vi "SoundMeasure.vi"() -> ()   [LabVIEW 2016]
uses:
  <vilib>/Instr/_visa.llb/VISA Configure Serial Port (Instr).vi
  <vilib>/Utility/config.llb/Read Key (Double).vi
  <vilib>/Utility/file.llb/Write Delimited Spreadsheet (DBL).vi
  <vilib>/Utility/config.llb/NI_LVConfig.lvlib
panel:
  in  "record cycle":u64=7 min=6 step=1
  in  "freq (MHz)":dbl=1.367 min=0.1 max=10.0 step=0.01
  in  "SETVOLT":bool
  out "error out":errorcluster
  in  "cycle":u32=120
  in  "Channel":u16
  in  "KYCT axis in HIFU coordinate":cluster{"X axis":dbl[], "Z axis":dbl[]}={"X axis"=[1.0, 0.0, 0.0], "Z axis"=[0.0, 0.0, 1.0]}
  in  "KYCT coordinate":T1
  in  "Sens (V/MPa)":dbl=0.1
  in  "Port":u32=12321
  in  "HIFU_connect":bool
  in  "HIFU_Telnet":bool
  out "Pressure (MPa)":dbl format="%#_4g"
  in  "pout":bool
  in  "totle chnnum":i16=64
  in  "HIFU IP":string="192.168.1.24"
  in  "SETPHS":bool
  out "XY Graph 2":T2(graph)
  in  "Set global voltage":bool
  in  "Voltage":dbl=4.0 min=0.5 max=20.0 step=1.0
  out "Sonication":bool
  in  "continuousOut":bool
  in  "Scan":bool
  in  "Tab Control":enum32{"1D Scan", "2D Scan", "Monitor"}(tab)
  out "1D plot":cluster{dbl[], dbl[]}(graph)
  out "2D Scan":dbl[][](graph)
  in  "start":bool
  in  "reord":bool
  out "Current":dbl[](graph)
  out "Voltage":dbl[](graph)
  in  "Go":bool
  in  "Speed":dbl=0.5 min=0.2 max=2.5 step=0.1
  in  "Position":dbl[](array[numeric]) format="%#_6f"
  in  "Z+":bool
  in  "Z-":bool
  in  "Y+":bool
  in  "Y-":bool
  in  "X+":bool
  in  "X-":bool
  in  "error in (no error)":errorcluster
  out "HIFU":bool
  out "osc":bool
  out "KYCT":bool
  in  "Exit":bool
  in  "3D motorized stage":refnum<visa-resource-name>
  in  "oscilloscope":refnum<visa-resource-name>
  # "Z"
  # "X"
  # "Y"
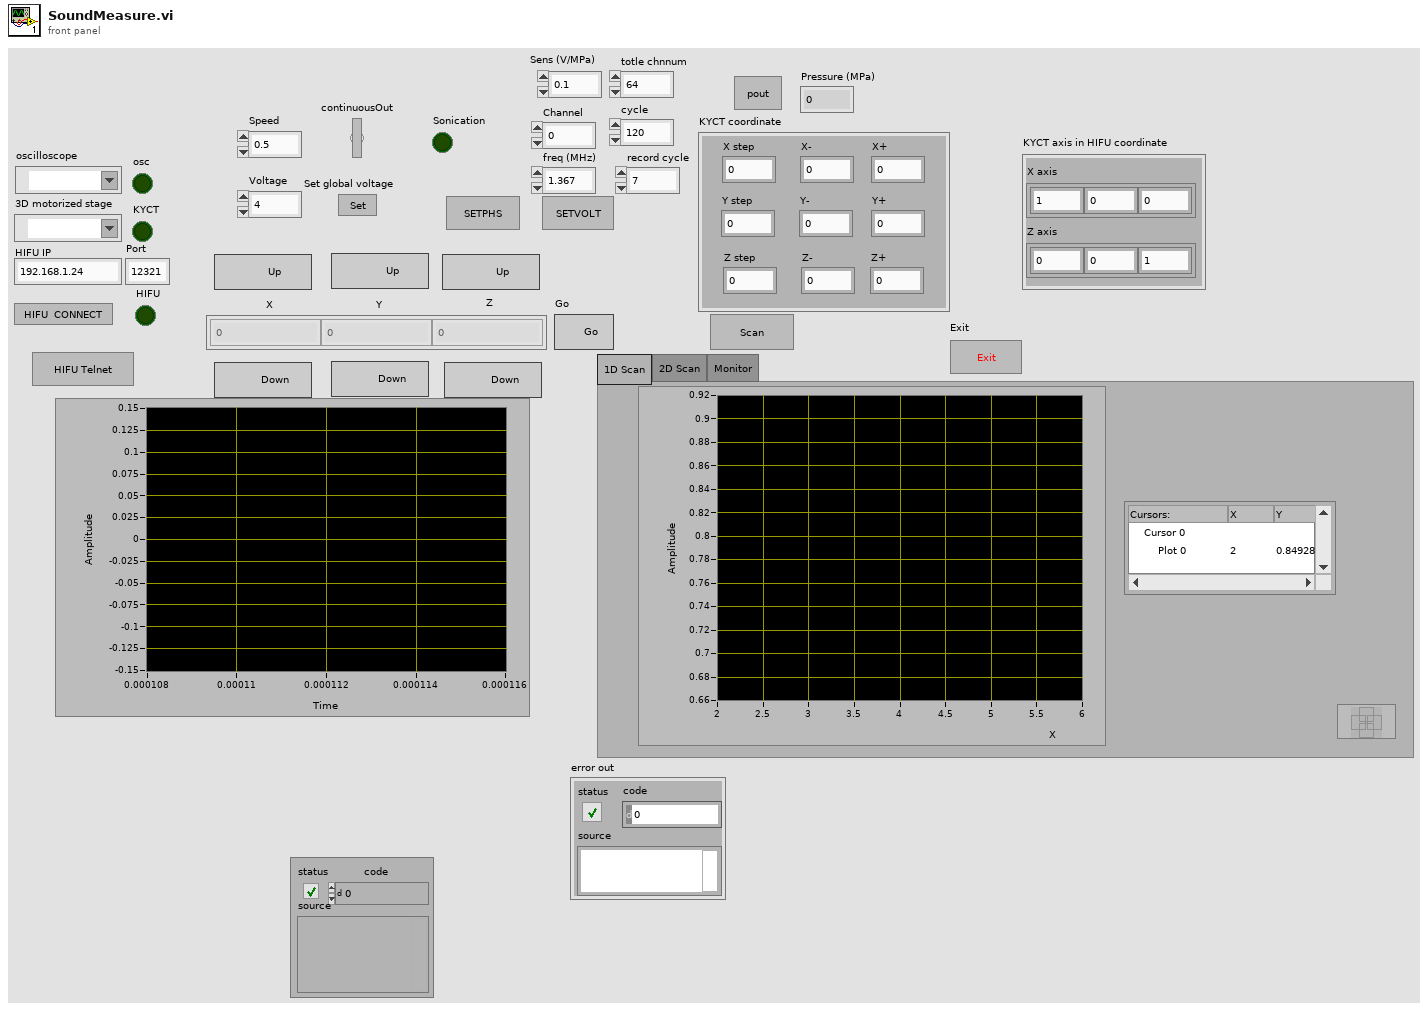
[diagram p1: front panel]
types:
  T1 = cluster{"X-":dbl, "X step":dbl, "Y-":dbl, "Y step":dbl, "Z-":dbl, "Z step":dbl, "Z+":dbl, "X+":dbl, "Y+":dbl}
  T2 = cluster{"time sequence":dbl[], "Voltage sequence":dbl[]}
  T3 = enum8{"Enabled", "Disabled", "Disabled and Grayed Out"}
  T4 = typedef "NI_LVConfig.lvlib/Config Data RefNum.ctl" = refnum<k1>
  T5 = typedef "NI_Matrix.lvlib/RealMatrix.ctl" = dbl[][]
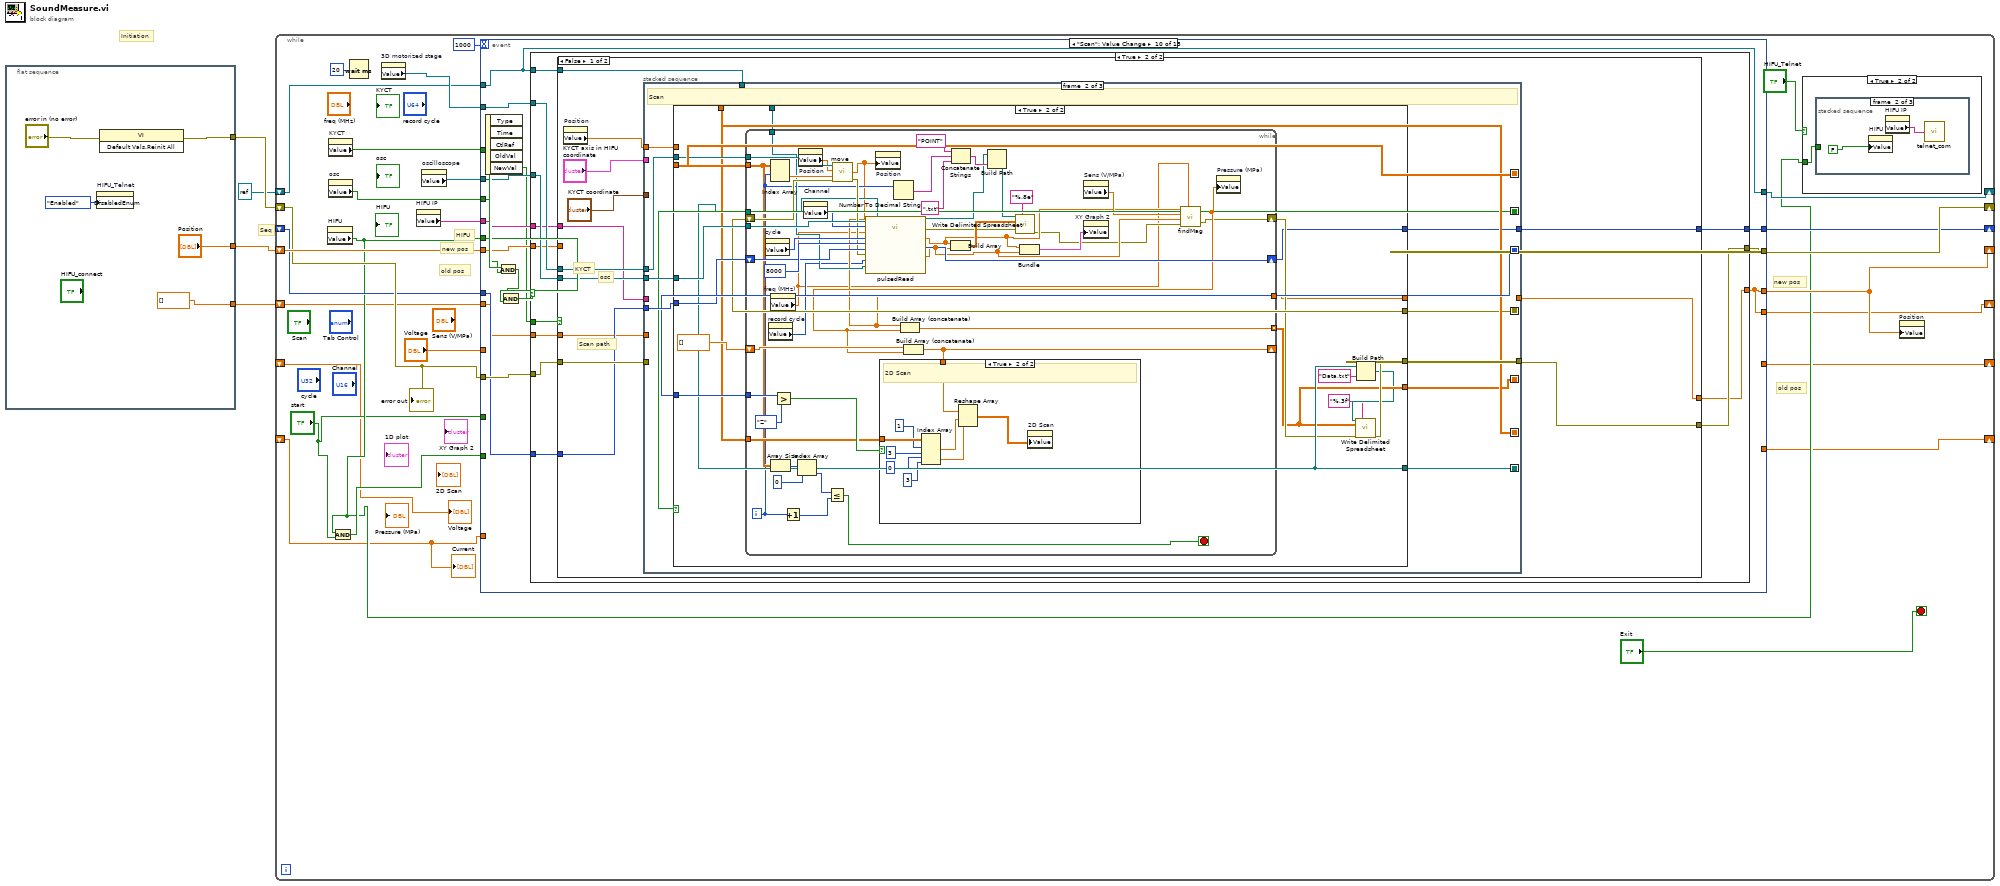
[diagram p0: block diagram]
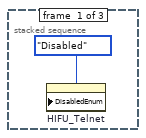
[diagram p3: hidden frame]
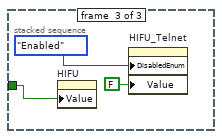
[diagram p4: hidden frame]
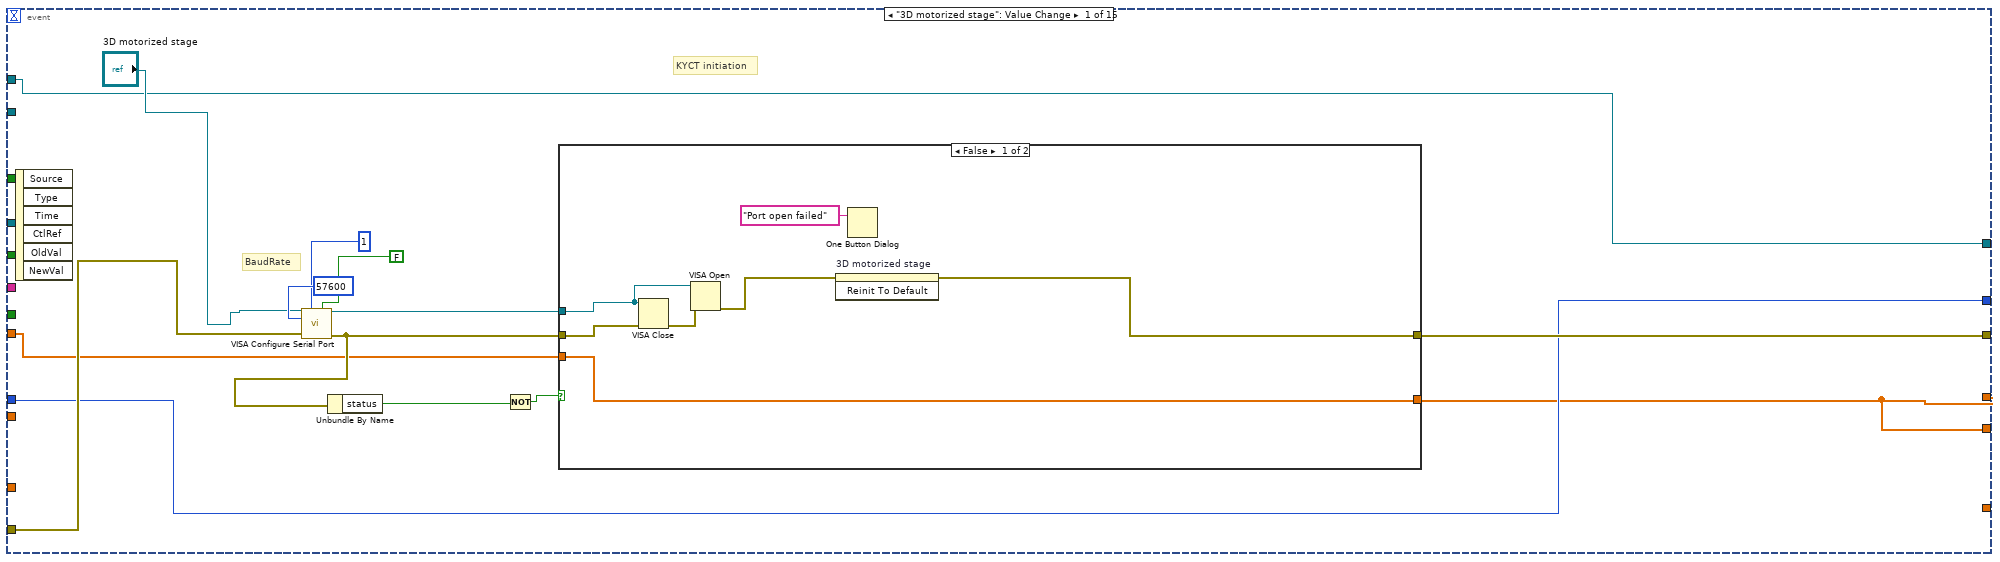
[diagram p5: hidden frame]
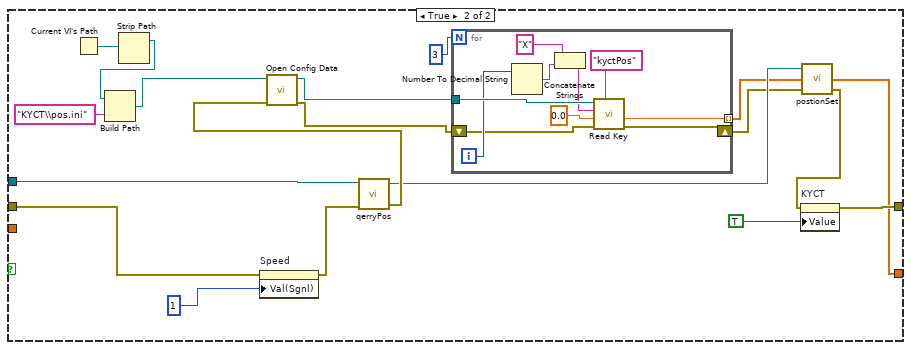
[diagram p6: hidden frame]
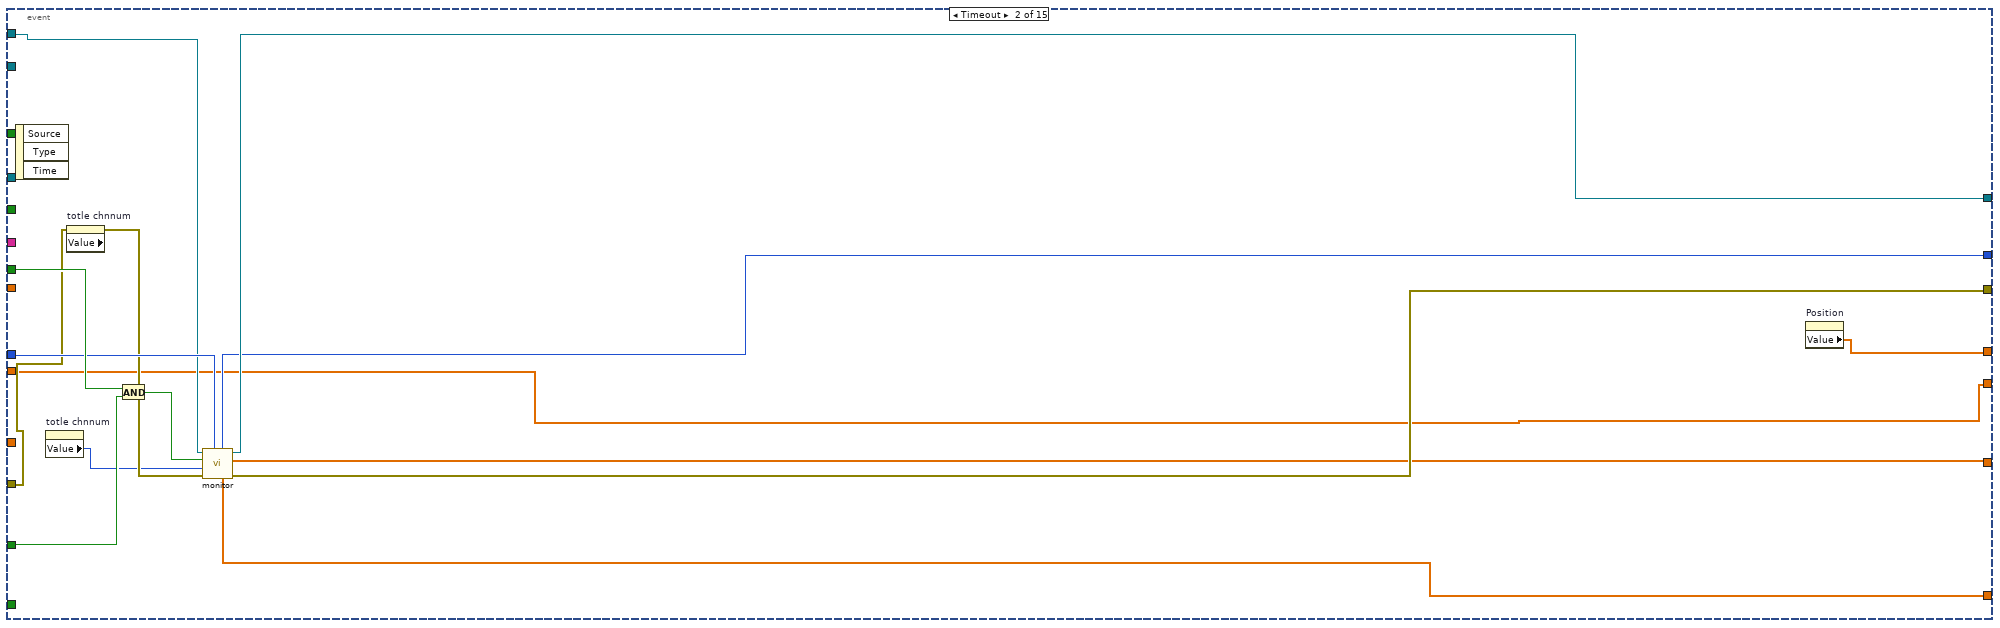
[diagram p7: hidden frame]
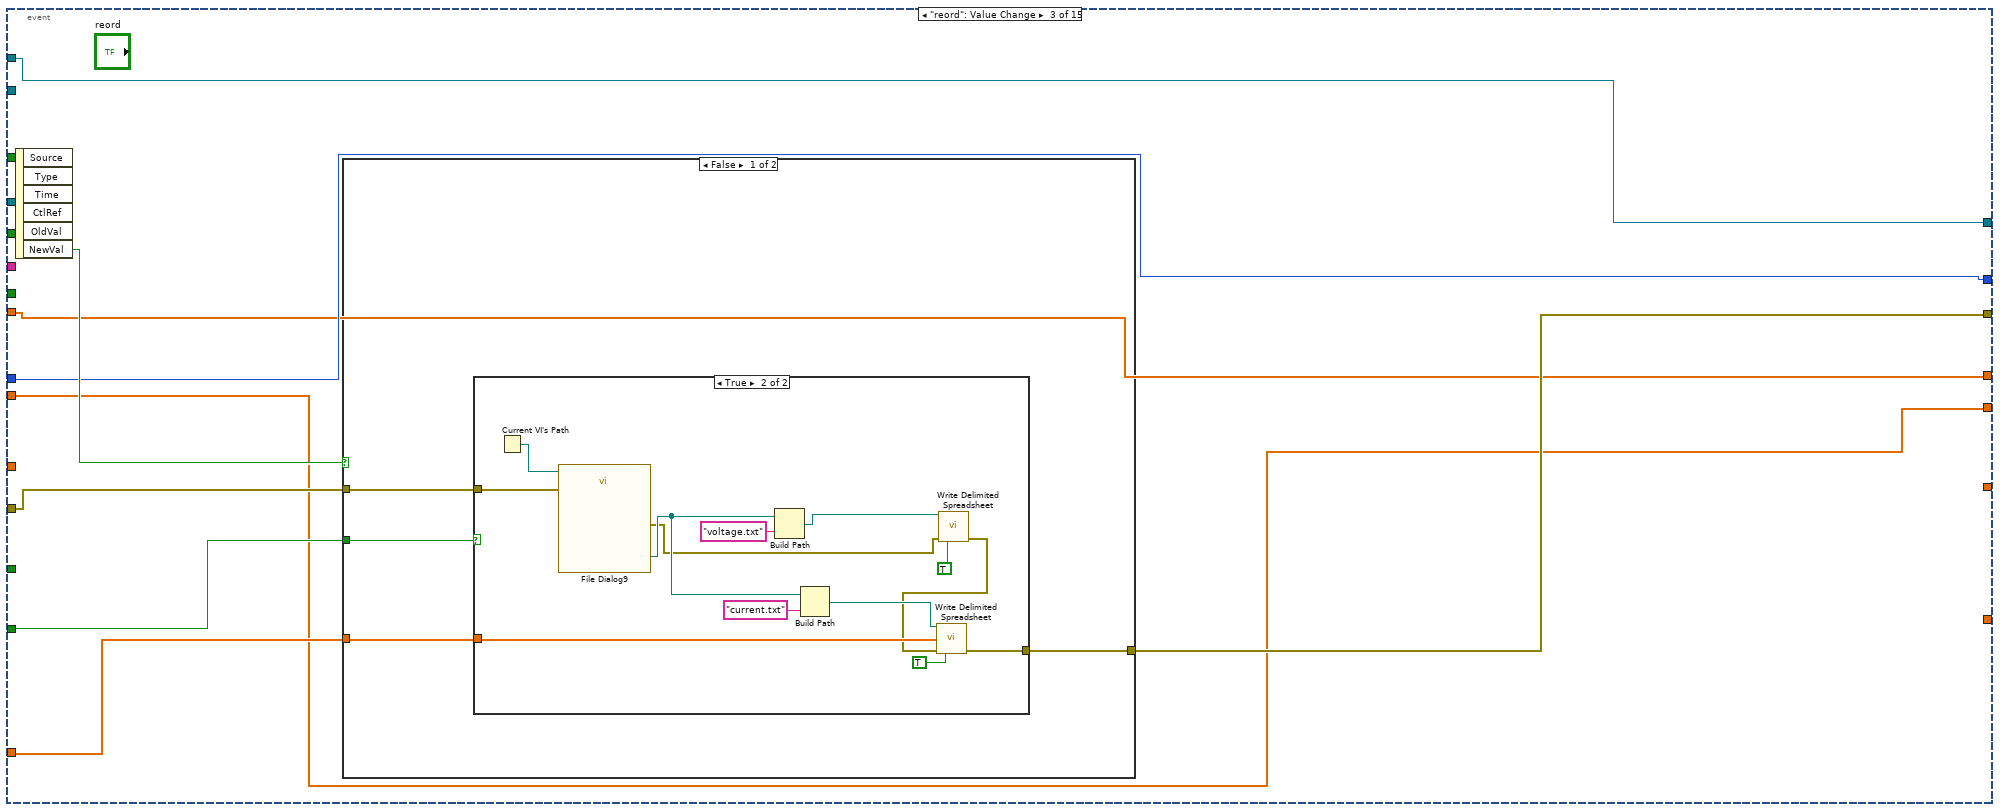
[diagram p8: hidden frame]
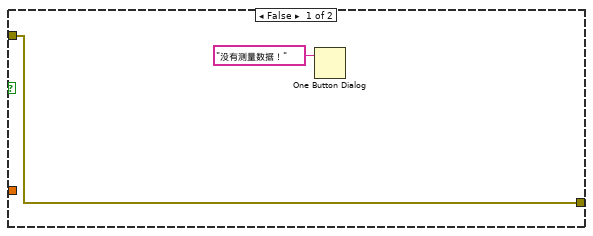
[diagram p9: hidden frame]
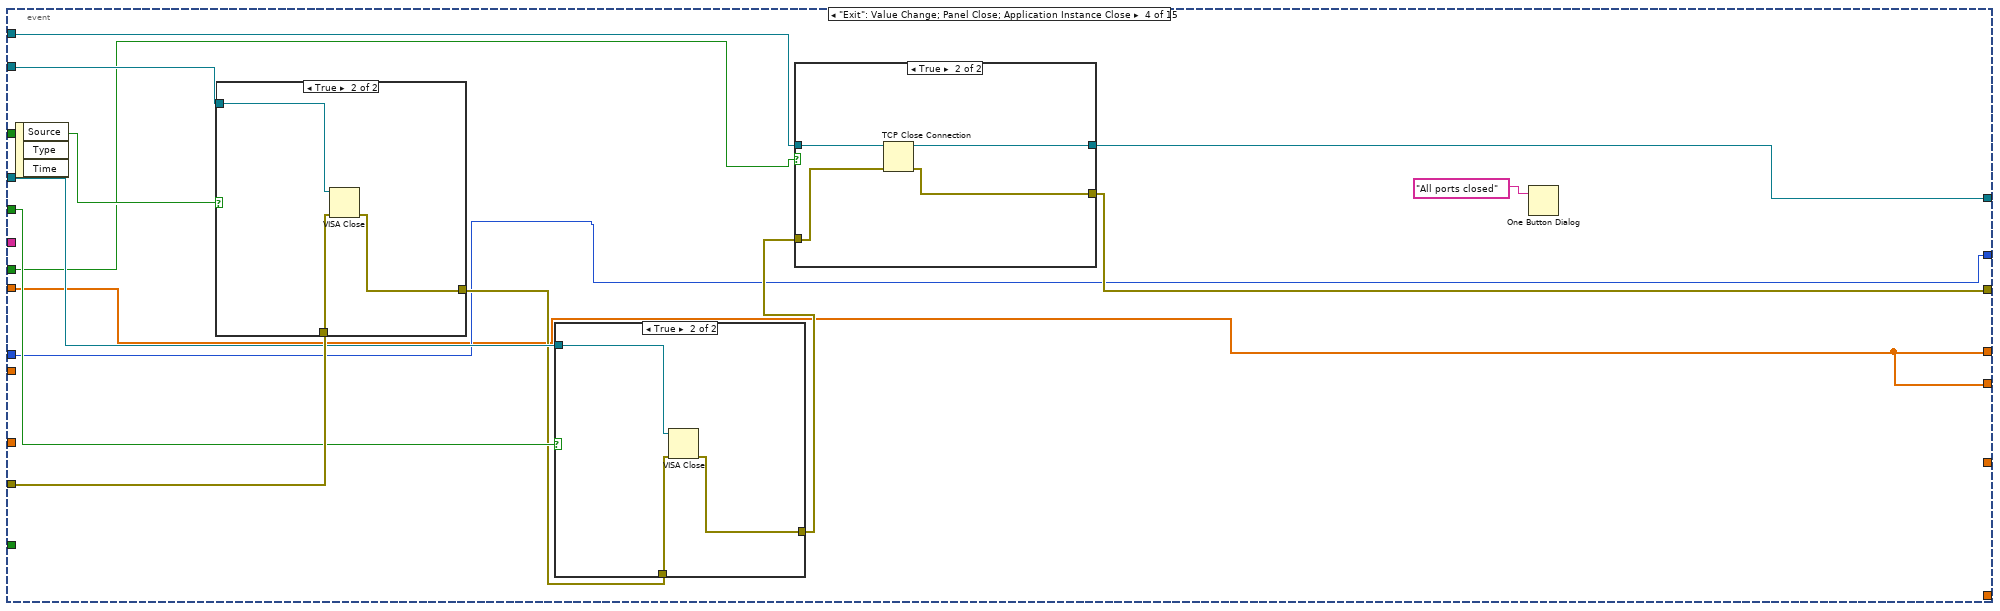
[diagram p11: hidden frame]
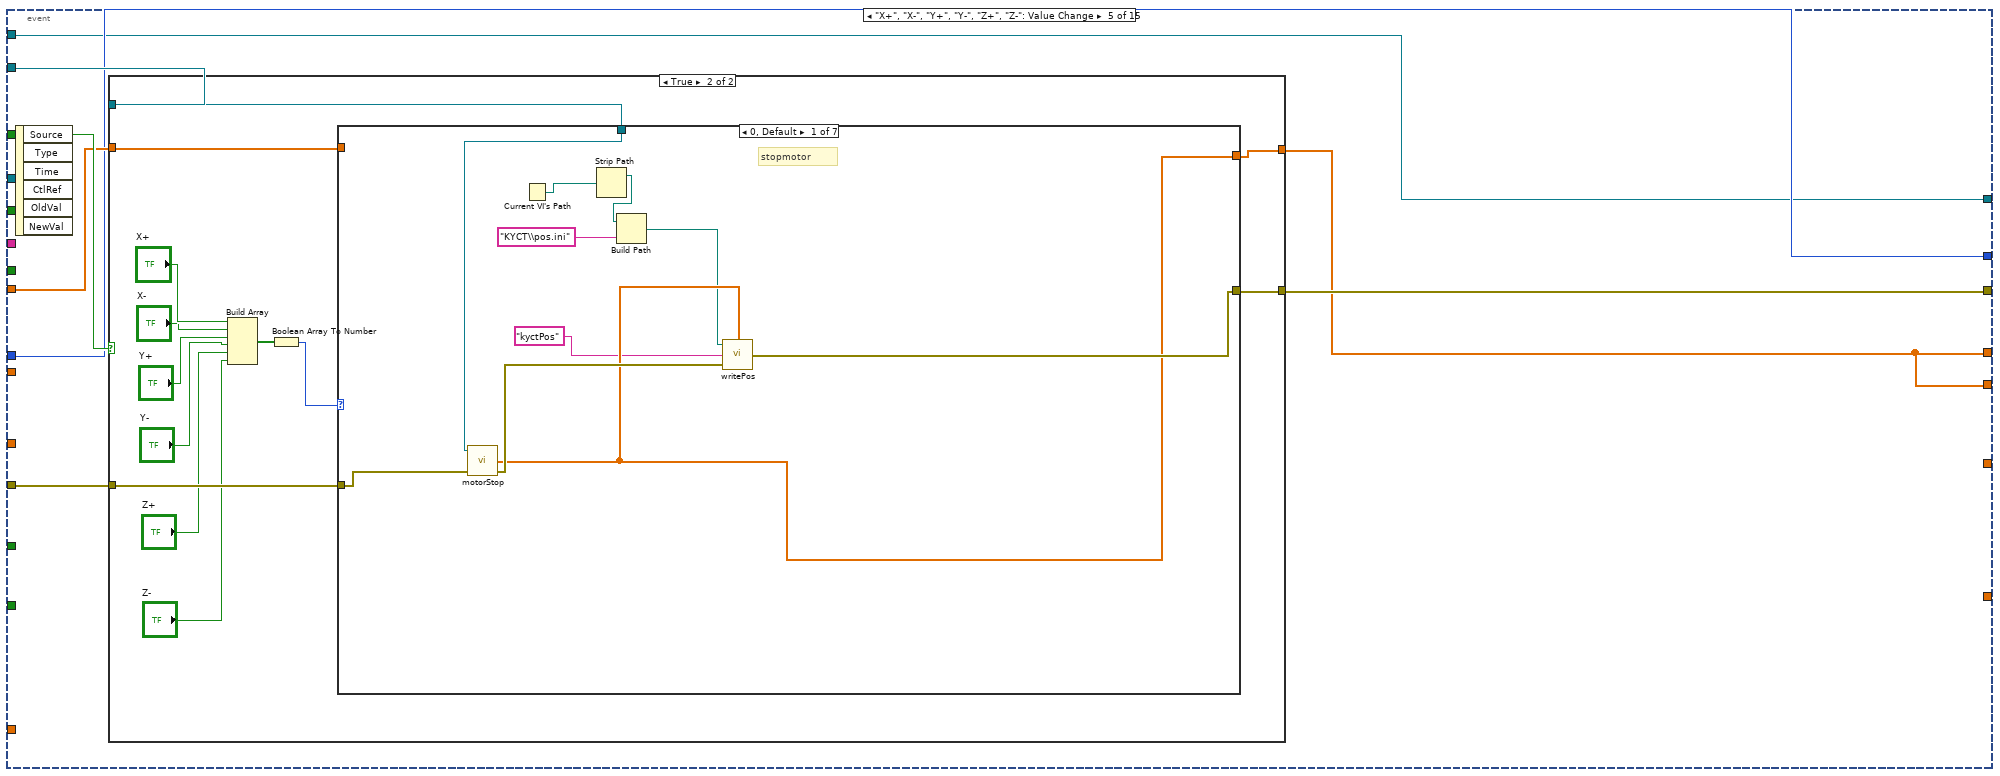
[diagram p15: hidden frame]
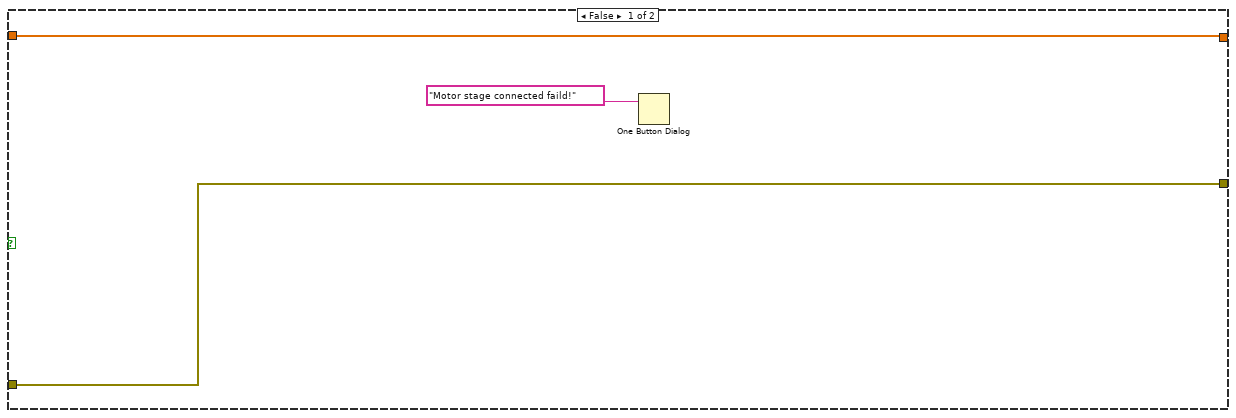
[diagram p16: hidden frame]
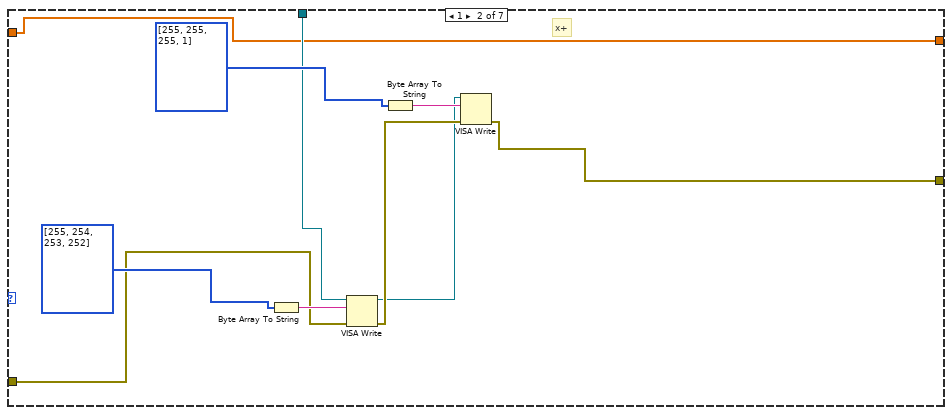
[diagram p17: hidden frame]
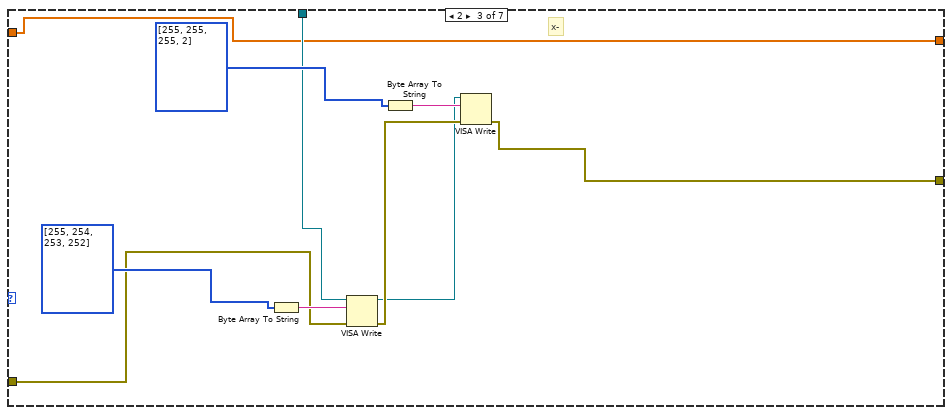
[diagram p18: hidden frame]
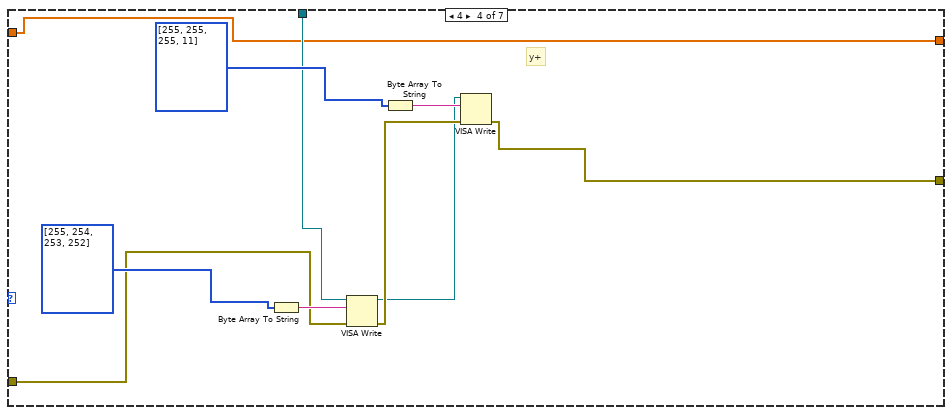
[diagram p19: hidden frame]
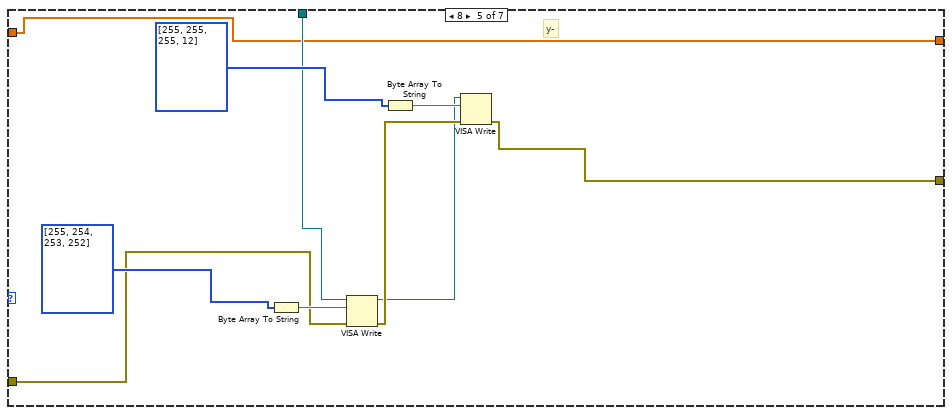
[diagram p20: hidden frame]
diagram:
  # "Seq"
  # "Initiation"
  n1 = flat-sequence {
    tunnel: ["Position"] -> w4
    tunnel: [w8] -> w3
    tunnel: [dbl[] []] -> w1
    frame #0 {
      n2 = property on="HIFU_Telnet" class="Bool (strict)"("DisabledEnum"=T3."Enabled" ("Disabled")) -> ()  [unwired: 2 in, 2 out]
      n3 = invoke class="VI" method="Default Vals.Reinit All"(error in="error in (no error)") -> (error out=w8:errorcluster)  [unwired: 2 in, 2 out]
    }
  }
  n4 = while {
    shift-right: [w34] -> _
    shift-left: w4 -> [w33]
    shift-right: [w32] -> _
    shift-left: w3 -> [w20]
    shift-right: [w23] -> _
    shift-left: refnum<k5> refnum ("connection ID out") -> [w22]
    shift-right: [w21] -> _
    shift-left: _ -> [w19]
    shift-right: [w17] -> _
    shift-left: _ -> [w16]
    shift-right: [w13] -> _
    shift-left: w1 -> [w12]
    shift-right: [w11] -> _
    shift-left: _ -> [w10]
    stop <- "Exit" stop-if-true
    # "HIFU"
    # "old pos"
    # "new pos"
    # "old pos"
    # "new pos"
    n5 = property on="HIFU" class="Bool (strict)"() -> ("Value"=w18:bool)  [unwired: 2 in, 2 out]
    n6 = property on="KYCT" class="Bool (strict)"() -> ("Value"=w36:bool)  [unwired: 2 in, 2 out]
    n7 = property on="osc" class="Bool (strict)"() -> ("Value"=w35:bool)  [unwired: 2 in, 2 out]
    n8 = And(x=w18, y="start") -> (x .and. y?=w25:bool)
    n9 = Wait (ms)(milliseconds to wait=u32 20) -> ()  [unwired: 1 out]
    n10 = property on="3D motorized stage" class="VISAName"() -> ("Value"=w30:refnum<visa-resource-name>)  [unwired: 2 in, 2 out]
    n11 = property on="HIFU IP" class="Str"() -> ("Value"=w26:string)  [unwired: 2 in, 2 out]
    n12 = property on="oscilloscope" class="VISAName"() -> ("Value"=w29:refnum<visa-resource-name>)  [unwired: 2 in, 2 out]
    n13 = event shown="[9] \"Scan\": Value Change" {
      selector: _ -> [_ _ _ _ _ _ _ _ _ _ _ _ _ _ _]
      dyn-events: _ -> [_ _ _ _ _ _ _ _ _ _ _ _ _ _ _]
      timeout: 1000 -> [_ _ _ _ _ _ _ _ _ _ _ _ _ _ _]
      tunnel: w30 -> [_ _ _ w150 w172 w267 w287 _ _ w403 _ _ _ _ _]
      tunnel: w29 -> [_ _ _ w147 _ _ _ _ _ w401 w638 _ _ _ _]
      tunnel: w20 -> [w53 w106 w117 w149 w171 w268 w286 w317 w358 w402 w637 w673 w683 w722 w752]
      tunnel: w36 -> [_ _ _ w151 w173 w266 w288 _ _ w408 _ _ _ _ w756]
      tunnel: [w55 w98 w115 w141 w170 w264 w284 w315 w356 w400 w636 w672 w681 w721 w751] -> w32
      tunnel: w35 -> [_ _ _ w148 _ _ _ _ _ w407 w635 _ _ _ _]
      tunnel: w33 -> [w48 _ w110 w138 w169 w261 _ w318 w359 w399 w639 w674 w684 w719 w755]
      tunnel: [w44 w96 w110 w138 w166 w261 w279 w318 w359 w393 w639 w674 w684 w719 w754] -> w34
      tunnel: w18 -> [_ w108 _ w144 _ _ _ w316 w357 w406 w634 _ _ w718 w749]
      tunnel: "Voltage" -> [_ _ _ _ _ _ _ _ _ _ _ _ _ w720 _]
      tunnel: w16 -> [_ _ w116 _ _ _ _ _ _ _ _ _ _ _ _]
      tunnel: w26 -> [_ _ _ _ _ _ _ _ _ w398 _ _ _ _ w748]
      tunnel: w25 -> [_ _ w114 _ _ _ _ _ _ _ _ _ _ _ _]
      tunnel: [w46 w102 w112 w139 w167 w262 w281 w313 w354 w394 w629 w669 w679 w714 w744] -> w23
      tunnel: w22 -> [w46 w103 w112 w142 w167 w262 w281 w313 w354 w394 w629 w669 _ w714 w747]
      tunnel: [w45 w100 w111 w140 w168 w263 w282 w311 w352 w395 w630 w670 w678 w715 w745] -> w21
      tunnel: w19 -> [w45 w107 w111 w140 w168 w263 w282 w312 w353 w396 w631 w670 _ w716 w746]
      tunnel: [_ w101 _ _ _ _ _ _ _ _ _ _ _ _ _] -> w17
      tunnel: "start" -> [_ w99 _ _ _ _ _ _ _ _ _ _ _ _ _]
      tunnel: [w44 w95 w109 w138 w166 w260 w278 w310 w351 w393 w628 w668 w677 w713 w743] -> w13
      tunnel: w12 -> [_ w95 w109 _ _ w260 w280 w310 w351 w392 w628 w668 w677 w713 w743]
      tunnel: [_ w94 _ _ _ _ _ _ _ _ _ _ _ _ _] -> w11
      event "3D motorized stage": Value Change {
        # "KYCT initiation"
        # "BaudRate"
        n14 = event-data() -> ()  [unwired: 1 in, 6 out]
        n15 = call-poly "VISA Configure Serial Port"("VISA resource name"="3D motorized stage", "timeout (10sec)"=u32 1, "Enable Termination\nChar (T)"=FALSE, "baud rate (9600)"=u32 57600, "error in (no error)"=w53) -> ("VISA resource name out"=w56:refnum<visa-resource-name>, "error out"=w51:errorcluster)  [unwired: 9 in]
        n16 = Unbundle By Name(w51) -> ("status"=w50:bool)
        n17 = Not(x=w50) -> (.not. x?=w49:bool)
        n18 = case shown="False" w49 {
          tunnel: w56 -> [w58 w81]
          tunnel: [w64 w66] -> w44
          tunnel: [w63 w80] -> w55
          tunnel: w51 -> [w61 w78]
          tunnel: w48 -> [w64 _]
          frame False {
            n19 = VISA Close(VISA resource name=w58, error in (no error)=w61) -> (error out=w60:errorcluster)
            n20 = VISA Open(error in (no error)=w60, VISA resource name=w58) -> (error out=w59:errorcluster)  [unwired: 3 in, 1 out]
            n21 = invoke on="3D motorized stage" class="VISAName" method="Reinit To Default"(error in=w59) -> (error out=w63:errorcluster)  [unwired: 2 in, 2 out]
            n22 = One Button Dialog(message="Port open failed") -> ()  [unwired: 1 in, 1 out]
          }
          frame True {
            n23 = Current VI's Path() -> (path=w77:path)
            n24 = Strip Path(path=w77) -> (stripped path=w76:path)  [unwired: 1 out]
            n25 = Build Path(base path=w76, name or relative path="KYCT\\pos.ini") -> (appended path=w74:path)
            n26 = property on="Speed" class="DigNum (strict)"(error in=w78, "Val(Sgnl)"=1) -> (error out=w79:errorcluster)  [unwired: 1 in, 1 out]
            n27 = call "qerryPos.vi"("error in (no error)"=w79, "UART in"=w81) -> ("error out"=w73:errorcluster, "UART out"=w69:refnum<visa-resource-name>)  [unwired: 2 in, 1 out]
            n28 = call <vilib>:"Open Config Data.vi"("error in (no error)"=w73, "configuration file path"=w74) -> ("error out"=w71:errorcluster, "refnum"=w70:T4)  [unwired: 7 in, 1 out]
            n29 = for {
              N: 3 -> [_]
              tunnel: w70 -> [w93]
              shift-right: [w86] -> w68
              shift-left: w71 -> [w87]
              tunnel: [w85] -> w67 mode=indexing
              i -> [w89]
              n30 = Number To Decimal String(number=w89) -> (decimal integer string=w91:string)  [unwired: 1 in]
              n31 = Concatenate Strings("X" ("string"), w91) -> (w90:string)
              n32 = call-poly <vilib>:"Read Key.vi"("section"="kyctPos", "error in (no error)"=w87, "default value"=0.0, "key"=w90, "refnum"=w93) -> ("error out"=w86:errorcluster, "value"=w85:dbl)  [unwired: 3 in, 2 out]
            }
            n33 = call "postionSet.vi"("error in (no error)"=w68, "Pos in"=w67, "UART PORT in"=w69) -> ("error out"=w65:errorcluster, "Pos out"=w66:dbl[])  [unwired: 1 out]
            n34 = property on="KYCT" class="Bool (strict)"(error in=w65, "Value"=TRUE) -> (error out=w80:errorcluster)  [unwired: 1 in, 1 out]
          }
        }
      }
      event Timeout {
        n35 = event-data() -> ()  [unwired: 1 in, 3 out]
        n36 = property on="totle chnnum" class="DigNum (strict)"() -> ("Value"=w97:i16)  [unwired: 2 in, 2 out]
        n37 = property on="totle chnnum" class="DigNum (strict)" props=["Value"](error in=w106) -> (error out=w105:errorcluster)  [unwired: 1 in, 2 out]
        n38 = And(x=w108, y=w99) -> (x .and. y?=w104:bool)
        n39 = call "monitor.vi"("HIFU_TCP in"=w103, "HIFU"=w104, "chn num"=w97, "error in (no error)"=w105, "sequence"=w107) -> ("SEQ out"=w100:u32, "current"=w101:dbl[], "HIFU_TCP out"=w102:refnum<k5>, "voltage"=w94:dbl[], "error out"=w98:errorcluster)  [unwired: 1 out]
        n40 = property on="Position" class="Arr (strict)"() -> ("Value"=w96:dbl[])  [unwired: 2 in, 2 out]
      }
      event "reord": Value Change {
        n41 = event-data() -> ("NewVal"=w113:bool)  [unwired: 1 in, 5 out]
        n42 = case shown="False" w113 {
          tunnel: w117 -> [w121 w137]
          tunnel: w116 -> [w120 _]
          tunnel: [w119 w137] -> w115
          tunnel: w114 -> [w118 _]
          frame False {
            n43 = case shown="True" w118 {
              tunnel: w121 -> [w123 w131]
              tunnel: w120 -> [_ w128]
              tunnel: [w123 w126] -> w119
              frame False {
                n44 = One Button Dialog(message="没有测量数据！") -> ()  [unwired: 1 in, 1 out]
              }
              frame True {
                n45 = Current VI's Path() -> (path=w136:path)
                n46 = call "File Dialog9"("start path"=w136, "error in"=w131) -> ("selected path"=w133:path, "error out"=w130:errorcluster)  [unwired: 10 in, 2 out]
                n47 = Build Path(base path=w133, name or relative path="voltage.txt") -> (appended path=w132:path)
                n48 = Build Path(base path=w133, name or relative path="current.txt") -> (appended path=w129:path)
                n49 = call-poly <vilib>:"Write Delimited Spreadsheet.vi"("file path (dialog if empty)"=w132, "error in (no error)"=w130, "transpose? (no:F)"=TRUE) -> ("error out"=w127:errorcluster)  [unwired: 11 in, 1 out]
                n50 = call-poly <vilib>:"Write Delimited Spreadsheet.vi"("file path (dialog if empty)"=w129, "1D data"=w128, "error in (no error)"=w127, "transpose? (no:F)"=TRUE) -> ("error out"=w126:errorcluster)  [unwired: 10 in, 1 out]
              }
            }
          }
          frame True {
          }
        }
      }
      event "Exit": Value Change; Panel Close; Application Instance Close {
        n51 = event-data() -> ()  [unwired: 1 in, 3 out]
        n52 = case shown="True" w151 {
          tunnel: w150 -> [_ w165]
          tunnel: w149 -> [w162 w164]
          tunnel: [w162 w163] -> w146
          frame False {
          }
          frame True {
            n53 = VISA Close(VISA resource name=w165, error in (no error)=w164) -> (error out=w163:errorcluster)
          }
        }
        n54 = case shown="True" w148 {
          tunnel: w147 -> [_ w161]
          tunnel: w146 -> [w158 w160]
          tunnel: [w158 w159] -> w143
          frame False {
          }
          frame True {
            n55 = VISA Close(VISA resource name=w161, error in (no error)=w160) -> (error out=w159:errorcluster)
          }
        }
        n56 = case shown="True" w144 {
          tunnel: w143 -> [w153 w156]
          tunnel: w142 -> [w152 w157]
          tunnel: [w153 w155] -> w141
          tunnel: [w152 w154] -> w139
          frame False {
          }
          frame True {
            n57 = TCP Close Connection(connection ID=w157, error in (no error)=w156) -> (connection ID out=w154:refnum<k5>, error out=w155:errorcluster)  [unwired: 1 in]
          }
        }
        n58 = One Button Dialog(message="All ports closed") -> ()  [unwired: 1 in, 1 out]
      }
      event "X+", "X-", "Y+", "Y-", "Z+", "Z-": Value Change {
        n59 = event-data() -> ()  [unwired: 1 in, 6 out]
        n60 = case shown="True" w173 {
          tunnel: w172 -> [_ w188]
          tunnel: w171 -> [w175 w189]
          tunnel: [w175 w187] -> w170
          tunnel: [w174 w185] -> w166
          tunnel: w169 -> [w174 w186]
          frame False {
            n61 = One Button Dialog(message="Motor stage connected faild!") -> ()  [unwired: 1 in, 1 out]
          }
          frame True {
            n62 = Build Array("X+", "X-", "Y+", "Y-", "Z+", "Z-") -> (w178:bool[])
            n63 = Boolean Array To Number(Boolean array=w178) -> (number=w177:u32)
            n64 = case shown="0, Default" w177 {
              tunnel: w189 -> [w199 w205 w215 w225 w235 w245 w255]
              tunnel: w188 -> [w198 w204 w214 w224 w234 w244 w254]
              tunnel: [w196 w201 w211 w221 w231 w241 w251] -> w187
              tunnel: w186 -> [_ w200 w210 w220 w230 w240 w250]
              tunnel: [w195 w200 w210 w220 w230 w240 w250] -> w185
              frame 0, Default {
                # "stopmotor"
                n65 = call "motorStop.vi"("error in (no error)"=w199, "UART PORT in"=w198) -> ("error out"=w197:errorcluster, "P1"=w195:dbl[])  [unwired: 1 in, 1 out]
                n66 = Current VI's Path() -> (path=w193:path)
                n67 = Strip Path(path=w193) -> (stripped path=w192:path)  [unwired: 1 out]
                n68 = Build Path(base path=w192, name or relative path="KYCT\\pos.ini") -> (appended path=w191:path)
                n69 = call "writePos.vi"("Pos"=w195, "error in (no error)"=w197, "name"="kyctPos", "ini Path in"=w191) -> ("error out"=w196:errorcluster)
              }
              frame 1 {
                # "x+"
                n70 = Byte Array To String(unsigned byte array=i32[] [255, 254, 253, 252]) -> (string=w207:string)
                n71 = VISA Write(VISA resource name=w204, write buffer=w207, error in (no error)=w205) -> (VISA resource name out=w202:refnum<visa-resource-name>, error out=w203:errorcluster)  [unwired: 1 out]
                n72 = Byte Array To String(unsigned byte array=i32[] [255, 255, 255, 1]) -> (string=w209:string)
                n73 = VISA Write(VISA resource name=w202, write buffer=w209, error in (no error)=w203) -> (error out=w201:errorcluster)  [unwired: 2 out]
              }
              frame 2 {
                # "x-"
                n74 = Byte Array To String(unsigned byte array=i32[] [255, 254, 253, 252]) -> (string=w217:string)
                n75 = VISA Write(VISA resource name=w214, write buffer=w217, error in (no error)=w215) -> (VISA resource name out=w212:refnum<visa-resource-name>, error out=w213:errorcluster)  [unwired: 1 out]
                n76 = Byte Array To String(unsigned byte array=i32[] [255, 255, 255, 2]) -> (string=w219:string)
                n77 = VISA Write(VISA resource name=w212, write buffer=w219, error in (no error)=w213) -> (error out=w211:errorcluster)  [unwired: 2 out]
              }
              frame 4 {
                # "y+"
                n78 = Byte Array To String(unsigned byte array=i32[] [255, 254, 253, 252]) -> (string=w227:string)
                n79 = VISA Write(VISA resource name=w224, write buffer=w227, error in (no error)=w225) -> (VISA resource name out=w222:refnum<visa-resource-name>, error out=w223:errorcluster)  [unwired: 1 out]
                n80 = Byte Array To String(unsigned byte array=i32[] [255, 255, 255, 11]) -> (string=w229:string)
                n81 = VISA Write(VISA resource name=w222, write buffer=w229, error in (no error)=w223) -> (error out=w221:errorcluster)  [unwired: 2 out]
              }
              frame 8 {
                # "y-"
                n82 = Byte Array To String(unsigned byte array=i32[] [255, 254, 253, 252]) -> (string=w237:string)
                n83 = VISA Write(VISA resource name=w234, write buffer=w237, error in (no error)=w235) -> (VISA resource name out=w232:refnum<visa-resource-name>, error out=w233:errorcluster)  [unwired: 1 out]
                n84 = Byte Array To String(unsigned byte array=i32[] [255, 255, 255, 12]) -> (string=w239:string)
                n85 = VISA Write(VISA resource name=w232, write buffer=w239, error in (no error)=w233) -> (error out=w231:errorcluster)  [unwired: 2 out]
              }
              frame 16 {
                # "z+"
                n86 = Byte Array To String(unsigned byte array=i32[] [255, 254, 253, 252]) -> (string=w247:string)
                n87 = VISA Write(VISA resource name=w244, write buffer=w247, error in (no error)=w245) -> (VISA resource name out=w242:refnum<visa-resource-name>, error out=w243:errorcluster)  [unwired: 1 out]
                n88 = Byte Array To String(unsigned byte array=i32[] [255, 255, 255, 21]) -> (string=w249:string)
                n89 = VISA Write(VISA resource name=w242, write buffer=w249, error in (no error)=w243) -> (error out=w241:errorcluster)  [unwired: 2 out]
              }
              frame 32 {
                # "z-"
                n90 = Byte Array To String(unsigned byte array=i32[] [255, 254, 253, 252]) -> (string=w257:string)
                n91 = VISA Write(VISA resource name=w254, write buffer=w257, error in (no error)=w255) -> (VISA resource name out=w252:refnum<visa-resource-name>, error out=w253:errorcluster)  [unwired: 1 out]
                n92 = Byte Array To String(unsigned byte array=i32[] [255, 255, 255, 22]) -> (string=w259:string)
                n93 = VISA Write(VISA resource name=w252, write buffer=w259, error in (no error)=w253) -> (error out=w251:errorcluster)  [unwired: 2 out]
              }
            }
          }
        }
      }
      event "Speed": Value Change {
        n94 = event-data() -> ()  [unwired: 1 in, 6 out]
        n95 = case shown="False" w266 {
          tunnel: "Speed" -> [_ w276]
          tunnel: w268 -> [w270 w275]
          tunnel: w267 -> [_ w274]
          tunnel: [w270 w271] -> w264
          frame False {
            n96 = One Button Dialog(message="Motor stage connected faild!") -> ()  [unwired: 1 in, 1 out]
          }
          frame True {
            n97 = call "setVel.vi"("error in (no error)"=w275, "speed"=w276, "UART in"=w274) -> ("error out"=w273:errorcluster, "UART out"=w272:refnum<visa-resource-name>)
            n98 = property on="3D motorized stage" class="VISAName"(error in=w273, "Value"=w272) -> (error out=w271:errorcluster)  [unwired: 1 in, 1 out]
          }
        }
      }
      event "Go": Value Change {
        n99 = event-data() -> ("NewVal"=w283:bool)  [unwired: 1 in, 5 out]
        n100 = property on="Position" class="Arr (strict)"() -> ("Value"=w277:dbl[])  [unwired: 2 in, 2 out]
        n101 = case shown="True" w288 {
          tunnel: w287 -> [_ w300]
          tunnel: w286 -> [w291 w299]
          tunnel: [w290 w295] -> w279
          tunnel: [w291 w298] -> w285
          tunnel: w277 -> [w290 w296]
          tunnel: w283 -> [_ w297]
          tunnel: w280 -> [w289 w294]
          tunnel: [w289 w293] -> w278
          frame False {
            n102 = One Button Dialog(message="Motor stage connected faild!") -> ()  [unwired: 1 in, 1 out]
          }
          frame True {
            n103 = case shown="False" w297 {
              tunnel: w300 -> [w306 _]
              tunnel: w299 -> [w305 w309]
              tunnel: [w304 w309] -> w298
              tunnel: [w301 w308] -> w295
              tunnel: w296 -> [w303 w308]
              tunnel: w294 -> [w302 w307]
              tunnel: [w301 w307] -> w293
              frame False {
                n104 = call "move.vi"("error in (no error)"=w305, "P01"=w303, "P0"=w302, "UART PORT in"=w306) -> ("error out"=w304:errorcluster, "P1"=w301:dbl[])  [unwired: 1 out]
              }
              frame True {
              }
            }
          }
        }
        n105 = invoke on="Go" class="Bool" method="Reinit To Default"(error in=w285) -> (error out=w284:errorcluster)  [unwired: 2 in, 2 out]
      }
      event "SETPHS": Value Change {
        n106 = event-data() -> ("NewVal"=w314:bool)  [unwired: 1 in, 5 out]
        n107 = case shown="True" w316 {
          tunnel: w317 -> [w321 w326]
          tunnel: [w321 w327] -> w315
          tunnel: w314 -> [_ w325]
          tunnel: w313 -> [_ w324]
          tunnel: w312 -> [w319 w323]
          tunnel: [w319 w322] -> w311
          frame False {
            n108 = One Button Dialog(message="i2c connected failed") -> ()  [unwired: 1 in, 1 out]
          }
          frame True {
            n109 = case shown="False" w325 {
              tunnel: [w335 w350] -> w327
              tunnel: w326 -> [w334 w350]
              tunnel: w324 -> [w331 _]
              tunnel: w323 -> [w329 w349]
              tunnel: [w328 w349] -> w322
              frame False {
                n110 = call "File Dialog8"("error in"=w334) -> ("selected path"=w338:path, "error out"=w333:errorcluster)  [unwired: 11 in, 2 out]
                n111 = case shown="No Error" w333 {
                  selector: w333 -> [w339 w345]
                  tunnel: w338 -> [w342 _]
                  tunnel: [w341 w346] -> w337
                  tunnel: [w340 w344] -> w336
                  frame No Error {
                    n112 = call "readPHS.vi"("error in (no error)"=w339, "Path"=w342) -> ("error out"=w340:errorcluster, "Array"=w341:u8[])
                  }
                  frame Error {
                    n113 = call <vilib>:"Clear Errors.vi"("error in (no error)"=w345, "specific error code to clear (0: all)"=43) -> ("error out"=w344:errorcluster)  [unwired: 4 in, 1 out]
                    n114 = for {
                      N: 64 -> [_]
                      tunnel: [0] -> w346 mode=indexing
                    }
                  }
                }
                n115 = call "PhaseSet.vi"("相位输入"=w337, "HIFU"=TRUE, "error in (no error)"=w336, "chn num"="totle chnnum", "SeqNum"=w329, "connection ID in"=w331) -> ("error out"=w335:errorcluster, "SeqOUT"=w328:u32)  [unwired: 2 out]
              }
              frame True {
              }
            }
          }
        }
      }
      event "SETVOLT": Value Change {
        n116 = event-data() -> ("NewVal"=w355:bool)  [unwired: 1 in, 5 out]
        n117 = case shown="True" w357 {
          tunnel: w358 -> [w362 w367]
          tunnel: [w362 w368] -> w356
          tunnel: w355 -> [_ w366]
          tunnel: w354 -> [_ w365]
          tunnel: w353 -> [w360 w364]
          tunnel: [w360 w363] -> w352
          frame False {
            n118 = One Button Dialog(message="i2c connected failed") -> ()  [unwired: 1 in, 1 out]
          }
          frame True {
            n119 = case shown="False" w366 {
              tunnel: [w376 w391] -> w368
              tunnel: w367 -> [w375 w391]
              tunnel: w365 -> [w373 _]
              tunnel: w364 -> [w371 w390]
              tunnel: [w370 w390] -> w363
              frame False {
                n120 = call "File Dialog2"("error in"=w375) -> ("selected path"=w379:path, "error out"=w374:errorcluster)  [unwired: 11 in, 2 out]
                n121 = case shown="No Error" w374 {
                  selector: w374 -> [w380 w386]
                  tunnel: w379 -> [w383 _]
                  tunnel: [w382 w387] -> w378
                  tunnel: [w381 w385] -> w377
                  frame No Error {
                    n122 = call "readVoltFile.vi"("error in (no error)"=w380, "Path"=w383) -> ("error out"=w381:errorcluster, "Array"=w382:sgl[])
                  }
                  frame Error {
                    n123 = call <vilib>:"Clear Errors.vi"("error in (no error)"=w386, "specific error code to clear (0: all)"=43) -> ("error out"=w385:errorcluster)  [unwired: 4 in, 1 out]
                    n124 = for {
                      N: 64 -> [_]
                      tunnel: [0] -> w387 mode=indexing
                    }
                  }
                }
                n125 = property on="totle chnnum" class="DigNum (strict)"() -> ("Value"=w369:i16)  [unwired: 2 in, 2 out]
                n126 = call "VoltChnSet.vi"("相位输入"=w378, "HIFU"=TRUE, "error in (no error)"=w377, "chn num"=w369, "SeqNum"=w371, "connection ID in"=w373) -> ("error out"=w376:errorcluster, "SeqOUT"=w370:u32)  [unwired: 2 out]
              }
              frame True {
              }
            }
          }
        }
      }
      event "Scan": Value Change {
        n127 = event-data() -> ("NewVal"=w397:bool)  [unwired: 1 in, 4 out]
        n128 = And(x=w408, y=w407) -> (x .and. y?=w405:bool)
        n129 = And(x=w405, y=w406) -> (x .and. y?=w404:bool)
        n130 = case shown="True" w404 {
          tunnel: w403 -> [_ w423]
          tunnel: w402 -> [w411 w422]
          tunnel: w401 -> [_ w421]
          tunnel: [w411 w420] -> w400
          tunnel: [w410 w413] -> w393
          tunnel: w399 -> [w410 w414]
          tunnel: w398 -> [_ w419]
          tunnel: w397 -> [_ w418]
          tunnel: w394 -> [_ w417]
          tunnel: w396 -> [w409 w416]
          tunnel: [w409 w415] -> w395
          tunnel: w392 -> [_ w412]
          frame False {
          }
          frame True {
            n131 = case shown="False" w418 {
              tunnel: w423 -> [w435 _]
              tunnel: w422 -> [w434 w627]
              tunnel: w421 -> [w433 _]
              tunnel: [w426 w627] -> w420
              tunnel: w419 -> [w432 _]
              tunnel: w417 -> [w431 _]
              tunnel: w416 -> [w429 w626]
              tunnel: [w430 w626] -> w415
              tunnel: w414 -> [_ w625]
              tunnel: [w425 w625] -> w413
              tunnel: w412 -> [w424 _]
              frame False {
                # "Scan path"
                # "osc"
                # "KYCT"
                n132 = property on="Position" class="Arr (strict)"() -> ("Value"=w436:dbl[])  [unwired: 2 in, 2 out]
                n133 = stacked-sequence {
                  seq-local: [w439 _ _] -> [_ w511 w609]
                  seq-local: [w443 _ _] -> [_ w509 _]
                  seq-local: [w442 _ _] -> [_ w516 _]
                  seq-local: [w441 _ _] -> [_ w508 _]
                  seq-local: [w437 _ _] -> [_ w510 w608]
                  seq-local: [_ w506 _] -> [_ _ w613]
                  seq-local: [w438 _ _] -> [_ w504 w605]
                  tunnel: w436 -> [w447 w503 _]
                  tunnel: w435 -> [_ w515 w602]
                  tunnel: w434 -> [w445 _ _]
                  tunnel: w433 -> [_ w514 _]
                  tunnel: [_ w507 _] -> w426
                  tunnel: w432 -> [_ _ _]
                  tunnel: w431 -> [_ w512 _]
                  tunnel: w429 -> [_ w513 _]
                  tunnel: [_ w505 _] -> w430
                  tunnel: "KYCT coordinate" -> [w440 _ _]
                  tunnel: "KYCT axis in HIFU coordinate" -> [w448 _ _]
                  tunnel: [_ _ w601] -> w425
                  tunnel: w424 -> [_ _ w604]
                  frame #0 {
                    # "Creat Scan Path"
                    n134 = Current VI's Path() -> (path=w446:path)
                    n135 = call "File Dialog"("start path"=w446, "error in"=w445) -> ("selected path"=w443:path, "error out"=w444:errorcluster)  [unwired: 10 in, 2 out]
                    n136 = call "ScanPath.vi"("Scan parameters"=w440, "Axis parameters"=w448, "Position"=w447, "error in (no error)"=w444) -> ("Scanmode"=w439:enum16{"X", "Y", "Z", "YZ", "XZ", "XY"}, "ScanPath"=w442:T5, "Scan Ready"=w438:bool, "Ticks"=w437:dbl[][], "error out"=w441:errorcluster)
                    n137 = case shown="\"XZ\"" w439 {
                      tunnel: w440 -> [w454 w460 w466 w478 w490 w502]
                      frame "X" {
                        n138 = Unbundle By Name(w454) -> ("X step"=w450:dbl, "X+"=w449:dbl, "X-"=w451:dbl)
                        n139 = property on="1D plot" class="XYGraph (strict)"("XScale.Increment"=w450, "XScale.Maximum"=w449, "XScale.Minimum"=w451, "XScale.MinorInc"=w450, "XScale.RngStart"=w451, "XScale.NameLbl.Text"="X" ("X Scale.Name Label.Text")) -> ()  [unwired: 2 in, 2 out]
                        n140 = local write "Tab Control"(enum32{"1D Scan", "2D Scan", "Monitor"}."1D Scan" ("Tab Control")) -> ()
                      }
                      frame "Y" {
                        n141 = Unbundle By Name(w460) -> ("Y step"=w456:dbl, "Y+"=w455:dbl, "Y-"=w457:dbl)
                        n142 = property on="1D plot" class="XYGraph (strict)"("XScale.Increment"=w456, "XScale.Maximum"=w455, "XScale.Minimum"=w457, "XScale.MinorInc"=w456, "XScale.RngStart"=w457, "XScale.NameLbl.Text"="X" ("X Scale.Name Label.Text")) -> ()  [unwired: 2 in, 2 out]
                        n143 = local write "Tab Control"(enum32{"1D Scan", "2D Scan", "Monitor"}."1D Scan" ("Tab Control")) -> ()
                      }
                      frame "Z" {
                        n144 = Unbundle By Name(w466) -> ("Z step"=w462:dbl, "Z+"=w461:dbl, "Z-"=w463:dbl)
                        n145 = property on="1D plot" class="XYGraph (strict)"("XScale.Increment"=w462, "XScale.Maximum"=w461, "XScale.Minimum"=w463, "XScale.MinorInc"=w462, "XScale.RngStart"=w463, "XScale.NameLbl.Text"="X" ("X Scale.Name Label.Text")) -> ()  [unwired: 2 in, 2 out]
                        n146 = local write "Tab Control"(enum32{"1D Scan", "2D Scan", "Monitor"}."1D Scan" ("Tab Control")) -> ()
                      }
                      frame "YZ" {
                        n147 = Unbundle By Name(w478) -> ("Y step"=w470:dbl, "Y+"=w472:dbl, "Y-"=w471:dbl, "Z step"=w467:dbl, "Z+"=w469:dbl, "Z-"=w468:dbl)
                        n148 = Add(x=w472, y=w471) -> (x+y=w477:dbl)
                        n149 = Add(x=w469, y=w468) -> (x+y=w476:dbl)
                        n150 = property on="2D Scan" class="IntGraph (strict)"("XScale.Multiplier"=w470, "XScale.Offset"=w477, "YScale.Multiplier"=w467, "YScale.Offset"=w476, "XScale.Increment"=w470, "XScale.Maximum"=w472, "XScale.Minimum"=w471, "YScale.Increment"=w467, "YScale.Maximum"=w469, "YScale.Minimum"=w468, "XScale.NameLbl.Text"="Z" ("X Scale.Name Label.Text"), "YScale.NameLbl.Text"="Y" ("Y Scale.Name Label.Text")) -> ()  [unwired: 2 in, 2 out]
                        n151 = local write "Tab Control"(enum32{"1D Scan", "2D Scan", "Monitor"}."2D Scan" ("Tab Control")) -> ()
                      }
                      frame "XZ" {
                        n152 = Unbundle By Name(w490) -> ("X step"=w482:dbl, "X+"=w484:dbl, "X-"=w483:dbl, "Z step"=w479:dbl, "Z+"=w481:dbl, "Z-"=w480:dbl)
                        n153 = Add(x=w484, y=w483) -> (x+y=w489:dbl)
                        n154 = Add(x=w481, y=w480) -> (x+y=w488:dbl)
                        n155 = property on="2D Scan" class="IntGraph (strict)"("YScale.Multiplier"=w482, "YScale.Offset"=w489, "XScale.Multiplier"=w479, "XScale.Offset"=w488, "YScale.Increment"=w482, "YScale.Maximum"=w484, "YScale.Minimum"=w483, "XScale.Increment"=w479, "XScale.Maximum"=w481, "XScale.Minimum"=w480, "YScale.NameLbl.Text"="Z" ("X Scale.Name Label.Text"), "XScale.NameLbl.Text"="X" ("Y Scale.Name Label.Text")) -> ()  [unwired: 2 in, 2 out]
                        n156 = local write "Tab Control"(enum32{"1D Scan", "2D Scan", "Monitor"}."2D Scan" ("Tab Control")) -> ()
                      }
                      frame "XY" {
                        n157 = Unbundle By Name(w502) -> ("X step"=w494:dbl, "X+"=w496:dbl, "X-"=w495:dbl, "Y step"=w491:dbl, "Y+"=w493:dbl, "Y-"=w492:dbl)
                        n158 = Add(x=w496, y=w495) -> (x+y=w501:dbl)
                        n159 = Add(x=w493, y=w492) -> (x+y=w500:dbl)
                        n160 = property on="2D Scan" class="IntGraph (strict)"("YScale.Multiplier"=w494, "YScale.Offset"=w501, "XScale.Multiplier"=w491, "XScale.Offset"=w500, "YScale.Increment"=w494, "YScale.Maximum"=w496, "YScale.Minimum"=w495, "XScale.Increment"=w491, "XScale.Maximum"=w493, "XScale.Minimum"=w492, "YScale.NameLbl.Text"="Y" ("X Scale.Name Label.Text"), "XScale.NameLbl.Text"="X" ("Y Scale.Name Label.Text")) -> ()  [unwired: 2 in, 2 out]
                        n161 = local write "Tab Control"(enum32{"1D Scan", "2D Scan", "Monitor"}."2D Scan" ("Tab Control")) -> ()
                      }
                    }
                  }
                  frame #1 {
                    # "Scan"
                    n162 = case shown="True" w504 {
                      tunnel: w516 -> [_ w538]
                      tunnel: w515 -> [_ w537]
                      tunnel: w514 -> [_ w536]
                      tunnel: w513 -> [w520 w535]
                      tunnel: w512 -> [_ w534]
                      tunnel: w511 -> [_ w533]
                      tunnel: w510 -> [_ w531]
                      tunnel: w509 -> [_ w529]
                      tunnel: w508 -> [w519 w528]
                      tunnel: [w519 w526] -> w507
                      tunnel: [dbl[][] [] w525] -> w506
                      tunnel: [w520 w524] -> w505
                      tunnel: [w517 w523] -> _
                      tunnel: w503 -> [w517 _]
                      frame False {
                        # "wrong scan dimension"
                      }
                      frame True {
                        n163 = while {
                          tunnel: w538 -> [w548]
                          tunnel: w537 -> [w581]
                          tunnel: w536 -> [w579]
                          tunnel: w534 -> [w573]
                          shift-right: [w572] -> w524
                          shift-left: w535 -> [w576]
                          tunnel: w529 -> [w563]
                          tunnel: [w557] -> w525 mode=indexing
                          tunnel: w533 -> [w556]
                          shift-right: [w551] -> _
                          shift-left: dbl[] [] -> [w554]
                          tunnel: w531 -> [w552]
                          shift-right: [w550] -> w527
                          shift-left: w528 -> [w583]
                          tunnel: [w541] -> w523
                          i -> [w545]
                          stop <- w542 stop-if-true
                          n164 = property on="cycle" class="DigNum (strict)"() -> ("Value"=w578:u32)  [unwired: 2 in, 2 out]
                          n165 = property on="record cycle" class="DigNum (strict)"() -> ("Value"=w540:u64)  [unwired: 2 in, 2 out]
                          n166 = Index Array(array=w548, index (row)=w545) -> (element=w582:dbl[])  [unwired: 1 in]
                          n167 = property on="freq (MHz)" class="DigNum (strict)"() -> ("Value"=w539:dbl)  [unwired: 2 in, 2 out]
                          n168 = Array Size(array=w548) -> (size(s)=w547:i32[])
                          n169 = Greater?(x=w556, y=enum16{"X", "Y", "Z", "YZ", "XZ", "XY"}."Z" ("Scanmode")) -> (0:w555:bool)
                          n170 = Increment(x=w545) -> (x+1=w543:i32)
                          n171 = Index Array(array=w547, index=0) -> (element=w544:i32)
                          n172 = property on="Position" class="Arr (strict)"() -> ("Value"=w580:dbl[])  [unwired: 2 in, 2 out]
                          n173 = property on="Channel" class="DigNum (strict)"() -> ("Value"=w575:u16)  [unwired: 2 in, 2 out]
                          n174 = Less Or Equal?(x=w544, y=w543) -> (x <= y?=w542:bool)
                          n175 = call "move.vi"("error in (no error)"=w583, "P01"=w582, "P0"=w580, "UART PORT in"=w581) -> ("error out"=w574:errorcluster, "P1"=w541:dbl[])  [unwired: 1 out]
                          n176 = call "pulsedRead.vi"("osc in"=w579, "connection ID"=w573, "recCycles"=w540, "channel"=w575, "error in (no error)"=w574, "freq (MHz)"=w539, "cycles"=w578, "points"=u64 8000, "SEQ IN"=w576) -> ("error out"=w570:errorcluster, "voltage"=w559:dbl[], "SEQ OUT"=w572:u32, "time"=w560:dbl[])  [unwired: 1 in, 2 out]
                          n177 = property on="Position" class="Arr (strict)"("Value"=w541) -> ()  [unwired: 2 in, 2 out]
                          n178 = Number To Decimal String(number=w545) -> (decimal integer string=w568:string)  [unwired: 1 in]
                          n179 = Build Array(w560, w559) -> (w571:T5)
                          n180 = Concatenate Strings("POINT" ("string"), w568, ".txt" ("string")) -> (w565:string)
                          n181 = Build Path(base path=w563, name or relative path=w565) -> (appended path=w564:path)
                          n182 = call-poly <vilib>:"Write Delimited Spreadsheet.vi"("file path (dialog if empty)"=w564, "format (%.3f)"="%.8e", "2D data"=w571, "error in (no error)"=w570) -> ("error out"=w558:errorcluster)  [unwired: 10 in, 1 out]
                          n183 = Bundle("time"=w560, "voltage"=w559) -> (w562:cluster{"time":dbl[], "voltage":dbl[]})  [unwired: 1 in]
                          n184 = property on="Sens (V/MPa)" class="DigNum (strict)"() -> ("Value"=w561:dbl)  [unwired: 2 in, 2 out]
                          n185 = property on="XY Graph 2" class="XYGraph (strict)"("Value"=w562) -> ()  [unwired: 2 in, 2 out]
                          n186 = call "findMag.vi"("times"=w560, "sens"=w561, "voltages"=w559, "error in (no error)"=w558, "freq"=w539) -> ("magfound"=w553:dbl, "error out"=w550:errorcluster)
                          n187 = Build Array (concatenate)(w541, w553) -> (w557:dbl[])
                          n188 = Build Array (concatenate)(w554, w553) -> (w551:dbl[])
                          n189 = case shown="True" w555 {
                            tunnel: w552 -> [w591 w598]
                            tunnel: w551 -> [w590 w600]
                            frame False {
                              w589 = 0 ("index")
                              # "1D plot"
                              n190 = Array Size(array=w590) -> (size(s)=w586:i32)
                              n191 = Array Subset(array=w591, index (row)=w589, length (row)=1 ("length"), index (col)=w589, length (col)=w586) -> (w587:dbl[][])
                              n192 = Reshape Array(w587, w586) -> (w585:dbl[])
                              n193 = Bundle(w585, w590) -> (w584:cluster{dbl[], dbl[]})  [unwired: 1 in]
                              n194 = property on="1D plot" class="XYGraph (strict)"("Value"=w584) -> ()  [unwired: 2 in, 2 out]
                            }
                            frame True {
                              # "2D Scan"
                              n195 = Index Array(array=w598, index (row) #1=1 ("index (row)"), index (col) #1=3 ("disabled index (col)"), index (row) #2=0 ("index (row)"), index (col) #2=3 ("disabled index (col)")) -> (element #1=w593:dbl, element #2=w592:dbl)
                              n196 = Reshape Array(w600, w593, w592) -> (w599:dbl[][])
                              n197 = property on="2D Scan" class="IntGraph (strict)"("Value"=w599) -> ()  [unwired: 2 in, 2 out]
                            }
                          }
                          n198 = property on="Pressure (MPa)" class="DigNum (strict)"("Value"=w553) -> ()  [unwired: 2 in, 2 out]
                        }
                        n199 = Build Path(base path=w529, name or relative path="Data.txt") -> (appended path=w522:path)
                        n200 = call-poly <vilib>:"Write Delimited Spreadsheet.vi"("file path (dialog if empty)"=w522, "format (%.3f)"="%.3f", "2D data"=w525, "error in (no error)"=w527) -> ("error out"=w526:errorcluster)  [unwired: 10 in, 1 out]
                      }
                    }
                  }
                  frame #2 {
                    # "matlab display"
                    n201 = property on="Position" class="Arr (strict)"() -> ("Value"=w603:dbl[])  [unwired: 2 in, 2 out]
                    n202 = call "move.vi"("P01"=w604, "P0"=w603, "UART PORT in"=w602) -> ("P1"=w601:dbl[])  [unwired: 1 in, 2 out]
                    n203 = property on="Position" class="Arr (strict)"("Value"=w601) -> ()  [unwired: 2 in, 2 out]
                    n204 = Two Button Dialog(message="Create MATLAB figure?", 1:"NO" ("F button name (\"Cancel\")"), 2:"YES" ("T button name (\"OK\")")) -> (T button?=w607:bool)
                    n205 = And(x=w605, y=w607) -> (x .and. y?=w606:bool)
                    n206 = case shown="True" w606 {
                      tunnel: w613 -> [_ w618]
                      tunnel: w609 -> [_ w616]
                      tunnel: w608 -> [_ w614]
                      frame False {
                      }
                      frame True {
                        n207 = Greater?(x=w616, y=enum16{"X", "Y", "Z", "YZ", "XZ", "XY"}."Z" ("Scanmode")) -> (0:w617:bool)
                        n208 = case shown="True" w617 {
                          tunnel: w618 -> [w621 w624]
                          tunnel: w616 -> [w620 w622]
                          tunnel: w614 -> [w619 w623]
                          frame False {
                            # "1D Scan"
                            n209 = script code="% data=load('Data1.txt');\n% Ticks = [-20:0.5:20;-20:0.5:20];\n% ScanMode = 0;\n%% begin\nglobal data Ticks ScanMode\nfig = figure;\nresizefactor = 4;\nxvec = data(:,1);\nyvec = data(:,2);\nzvec = data(:,3);\nPvec = data(:,4);\nHIFUxvec = Ticks(1,:);\nh1 = plot(HIFUxvec,Pvec);\ndcm_obj = datacursormode(fig);\nset(dcm_obj,'UpdateFcn',@cursorfunc); \nswitch ScanMode\n    case 0\n        labelx = 'X in HIFU Coord (mm)';\n    case 1\n        labelx = 'Y in HIFU Coord (mm)';\n    case 2\n        labelx = 'Z in HIFU Coord (mm)';\nend\nxlabel(labelx);\nylabel('Acousctic pressure (MPa)');"("data"=w621, "ScanMode"=w620, "Ticks"=w619) -> ()  [unwired: 1 in, 1 out]
                          }
                          frame True {
                            # "2D Scan"
                            n210 = script code="% data=load('Data2.txt');\n% Ticks = [-15,1,15,31;-8,0.5,8,33];\n% ScanMode = 5;\n%% begin\nglobal data Ticks ScanMode\nfig = figure;\nresizefactor = 4;\nxvec = data(:,1);\nyvec = data(:,2);\nzvec = data(:,3);\nPvec = data(:,4);\nHIFUxvec = Ticks(1,1):Ticks(1,2):Ticks(1,3);\nHIFUyvec = Ticks(2,1):Ticks(2,2):Ticks(2,3);\nHIFUxnum = Ticks(1,4);\nHIFUynum = Ticks(2,4);\nPmap = reshape(Pvec,HIFUxnum,HIFUynum);%反过来\nh1 = imagesc(HIFUyvec,HIFUxvec,Pmap);%反过来\ndcm_obj = datacursormode(fig);\nset(dcm_obj,'UpdateFcn',@cursorfunc); \nswitch ScanMode\n    case 3\n        labely = 'Y in HIFU Coord (mm)';\n        labelx = 'Z in HIFU Coord (mm)';\n    case 4\n        labely = 'X in HIFU Coord (mm)';\n        labelx = 'Z in HIFU Coord (mm)';\n    case 5\n        labely = 'X in HIFU Coord (mm)';\n        labelx = 'Y in HIFU Coord (mm)';\nend\nxlabel(labelx);\nylabel(labely);\ncolormap('jet');\nhcb = colorbar;\nylabel(hcb,'Acousctic pressure (MPa)')"("data"=w624, "Ticks"=w623, "ScanMode"=w622) -> ()  [unwired: 1 in, 1 out]
                          }
                        }
                      }
                    }
                  }
                }
              }
              frame True {
              }
            }
          }
        }
      }
      event "pout": Value Change {
        n211 = event-data() -> ("NewVal"=w632:bool)  [unwired: 1 in, 5 out]
        n212 = And(x=w635, y=w634) -> (x .and. y?=w633:bool)
        n213 = case shown="False" w632 {
          tunnel: w638 -> [w646 _]
          tunnel: w637 -> [w645 w667]
          tunnel: [w644 w667] -> w636
          tunnel: w633 -> [w643 _]
          tunnel: w631 -> [w642 w666]
          tunnel: w629 -> [w641 _]
          tunnel: [w640 w666] -> w630
          frame False {
            n214 = case shown="True" w643 {
              tunnel: w646 -> [_ w665]
              tunnel: w645 -> [w649 w664]
              tunnel: [w649 w659] -> w644
              tunnel: w642 -> [w647 w658]
              tunnel: w641 -> [_ w657]
              tunnel: [w647 w656] -> w640
              frame False {
                n215 = One Button Dialog(message="HIFU或示波器没有连接！") -> ()  [unwired: 1 in, 1 out]
              }
              frame True {
                n216 = property on="record cycle" class="DigNum (strict)"() -> ("Value"=w651:u64)  [unwired: 2 in, 2 out]
                n217 = property on="freq (MHz)" class="DigNum (strict)"() -> ("Value"=w650:dbl)  [unwired: 2 in, 2 out]
                n218 = property on="Channel" class="DigNum (strict)"() -> ("Value"=w652:u16)  [unwired: 2 in, 2 out]
                n219 = property on="cycle" class="DigNum (strict)"() -> ("Value"=w653:u32)  [unwired: 2 in, 2 out]
                n220 = call "pulsedRead.vi"("osc in"=w665, "connection ID"=w657, "recCycles"=w651, "channel"=w652, "error in (no error)"=w664, "freq (MHz)"=w650, "cycles"=w653, "points"=u64 80000, "SEQ IN"=w658) -> ("error out"=w660:errorcluster, "voltage"=w661:dbl[], "SEQ OUT"=w656:u32, "time"=w662:dbl[])  [unwired: 1 in, 2 out]
                n221 = property on="pulsedRead.viSens (V/MPa)" class="DigNum (strict)"() -> ("Value"=w655:dbl)  [unwired: 2 in, 2 out]
                n222 = call "findMag.vi"("times"=w662, "sens"=w655, "voltages"=w661, "error in (no error)"=w660, "freq"=w650) -> ("magfound"=w654:dbl, "error out"=w659:errorcluster)
                n223 = property on="Pressure (MPa)" class="DigNum (strict)"("Value"=w654) -> ()  [unwired: 2 in, 2 out]
              }
            }
          }
          frame True {
          }
        }
      }
      event "oscilloscope": Value Change {
        # "Osc initiation"
        n224 = event-data() -> ()  [unwired: 1 in, 6 out]
        n225 = VISA Open(error in (no error)=w673, VISA resource name="oscilloscope") -> (error out=w675:errorcluster)  [unwired: 3 in, 1 out]
        n226 = property on="osc" class="Bool (strict)"(error in=w675, "Value"=TRUE) -> (error out=w672:errorcluster)  [unwired: 1 in, 1 out]
      }
      event "HIFU_connect": Value Change {
        n227 = event-data() -> ("NewVal"=w682:bool)  [unwired: 1 in, 5 out]
        n228 = case shown="False" w682 {
          tunnel: w683 -> [w686 w711]
          tunnel: [w691 w711] -> w681
          tunnel: [w690 FALSE] -> w680
          tunnel: [w688 refnum<k5> refnum ("connection ID")] -> w679
          tunnel: [w687 u32 0] -> w678
          frame False {
            n229 = call <vilib>:"Simple Error Handler.vi"("error in (no error)"=w686) -> ("error out"=w685:errorcluster)  [unwired: 4 in, 4 out]
            n230 = TCP Open Connection(address="HIFU IP", remote port or service name="Port", timeout ms (60000)=10000, error in (no error)=w685) -> (connection ID=w689:refnum<k5>, error out=w692:errorcluster)  [unwired: 1 in]
            n231 = case shown="No Error" w692 {
              selector: w692 -> [w698 w705]
              tunnel: [w698 w704] -> w691
              tunnel: [TRUE FALSE] -> w690
              tunnel: w689 -> [w697 _]
              tunnel: [w697 refnum<k5> refnum ("connection ID")] -> w688
              tunnel: [u32 0 u32 0] -> w687
              frame No Error {
              }
              frame Error {
                # "Timeout"
                n232 = Unbundle By Name(w705) -> ("code"=w706:i32)
                n233 = case shown="56" w706 {
                  tunnel: w705 -> [w707 _]
                  tunnel: [w707 w708] -> w704
                  frame Default {
                  }
                  frame 56 {
                    w708 = errorcluster {"status"=FALSE, "code"=0, "source"=""}  # No error
                  }
                }
                n234 = One Button Dialog(message="Connecting HIFU failed. Timeout.") -> ()  [unwired: 1 in, 1 out]
              }
            }
          }
          frame True {
          }
        }
        n235 = property on="HIFU" class="Bool (strict)"("Value"=w680) -> ()  [unwired: 2 in, 2 out]
      }
      event "Set global voltage": Value Change {
        n236 = event-data() -> ("NewVal"=w717:bool)  [unwired: 1 in, 5 out]
        n237 = case shown="False" w717 {
          tunnel: w722 -> [w729 w742]
          tunnel: [w728 w742] -> w721
          tunnel: w720 -> [w727 _]
          tunnel: w718 -> [w726 _]
          tunnel: w714 -> [w725 _]
          tunnel: w716 -> [w724 w741]
          tunnel: [w723 w741] -> w715
          frame False {
            n238 = case shown="True" w726 {
              tunnel: w729 -> [w731 w739]
              tunnel: [w731 w738] -> w728
              tunnel: w727 -> [_ w737]
              tunnel: w725 -> [_ w735]
              tunnel: w724 -> [w730 w734]
              tunnel: [w730 w733] -> w723
              frame False {
                n239 = One Button Dialog(message="i2c AMP connecting failed") -> ()  [unwired: 1 in, 1 out]
              }
              frame True {
                n240 = call "voltageSet.vi"("error in (no error)"=w739, "SEQ in"=w734, "Voltage"=w737, "connection ID"=w735) -> ("error out"=w738:errorcluster, "SEQ out"=w733:u32, "OK？"=w736:bool)  [unwired: 1 out]
                n241 = case shown="False" w736 {
                  frame True {
                  }
                  frame False {
                    n242 = One Button Dialog(message="Seting voltage failed") -> ()  [unwired: 1 in, 1 out]
                  }
                }
              }
            }
          }
          frame True {
          }
        }
      }
      event "continuousOut": Value Change {
        n243 = event-data() -> ()  [unwired: 1 in, 6 out]
        n244 = case shown="False" w756 {
          tunnel: w755 -> [_ w795]
          tunnel: [_ w795] -> w754
          frame False {
          }
          frame True {
          }
        }
        n245 = case shown="False" "continuousOut" {
          tunnel: [0 1] -> w753
          tunnel: [FALSE TRUE] -> _
          frame False {
          }
          frame True {
          }
        }
        n246 = case shown="True" w749 {
          tunnel: w753 -> [_ w761]
          tunnel: w752 -> [w759 w765]
          tunnel: [w759 w764] -> w751
          tunnel: w748 -> [_ _]
          tunnel: w747 -> [w757 w767]
          tunnel: w746 -> [w758 w766]
          tunnel: [w758 w763] -> w745
          tunnel: [w757 w762] -> w744
          frame False {
          }
          frame True {
            n247 = case shown="1" w761 {
              tunnel: w767 -> [w773 w788]
              tunnel: w766 -> [w774 w787]
              tunnel: w765 -> [_ w785]
              tunnel: [w770 w784] -> w764
              tunnel: [w771 w782] -> w763
              tunnel: [w772 w781] -> w762
              tunnel: [w768 w778] -> w760
              frame 0, Default {
                n248 = call "STOPheat.vi"("connection ID"=w773, "SEQ in"=w774) -> ("connection ID out"=w772:refnum<k5>, "SEQ out"=w771:u32, "OK?"=w769:bool, "error out"=w770:errorcluster)  [unwired: 1 in]
                n249 = case shown="True" w769 {
                  tunnel: [w775 FALSE] -> w768
                  frame False {
                    n250 = property on="Sonication" class="Bool (strict)"() -> ("Value"=w775:bool)  [unwired: 2 in, 2 out]
                  }
                  frame True {
                  }
                }
              }
              frame 1 {
                n251 = property on="totle chnnum" class="DigNum (strict)"() -> ("Value"=w786:i16)  [unwired: 2 in, 2 out]
                n252 = property on="Channel" class="DigNum (strict)"() -> ("Value"=w777:u16)  [unwired: 2 in, 2 out]
                n253 = call "PulsedOut.vi"("Cycles"=u64 360000000000000, "Channel"=w777, "frequency (MHz)"=1.367, "error in (no error)"=w785, "SEQ IN"=w787, "chn num"=w786, "connection ID"=w788) -> ("error out"=w784:errorcluster, "OK?"=w779:bool, "connection ID out"=w781:refnum<k5>, "SEQ OUT"=w782:u32)
                n254 = case shown="False" w779 {
                  tunnel: [w789 TRUE] -> w778
                  frame False {
                    n255 = property on="Sonication" class="Bool (strict)"() -> ("Value"=w789:bool)  [unwired: 2 in, 2 out]
                  }
                  frame True {
                  }
                }
              }
            }
            "Sonication" <- w760
          }
        }
      }
    }
    n256 = case shown="True" "HIFU_Telnet" {
      tunnel: w18 -> [_ w37]
      frame False {
      }
      frame True {
        n257 = stacked-sequence {
          tunnel: w37 -> [_ _ w41]
          frame #0 {
            n258 = property on="HIFU_Telnet" class="Bool (strict)"("DisabledEnum"=T3."Disabled" ("Disabled")) -> ()  [unwired: 2 in, 2 out]
          }
          frame #1 {
            n259 = property on="HIFU" class="Bool (strict)"("Value"=FALSE) -> ()  [unwired: 2 in, 2 out]
            n260 = property on="HIFU IP" class="Str"() -> ("Value"=w39:string)  [unwired: 2 in, 2 out]
            n261 = call "telnet_com.vi"("HIFU ip"=w39) -> ()
          }
          frame #2 {
            n262 = property on="HIFU" class="Bool (strict)"("Value"=w41) -> ()  [unwired: 2 in, 2 out]
            n263 = property on="HIFU_Telnet" class="Bool (strict)"("DisabledEnum"=T3."Enabled" ("Disabled"), "Value"=FALSE ("HIFU_Telnet")) -> ()  [unwired: 2 in, 2 out]
          }
        }
      }
    }
    n264 = property on="Position" class="Arr (strict)"("Value"=w34) -> ()  [unwired: 2 in, 2 out]
    "Current" <- w16
    "Voltage" <- w10
    "error out" <- w20
  }
